vi "BRig_dataCurrent_s_Selection.vi"() -> (2 "output_s_Selection":i32)   [LabVIEW 2014]
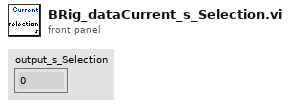
[diagram p1: front panel]
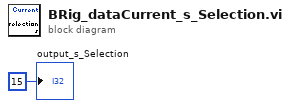
[diagram p0: block diagram]
diagram:
  "output_s_Selection" <- 15 ("output_iBlock")
